vi "_easyXML_Marshal.vi"   [LabVIEW 2013, in "OpenSerializer.easyXML.lvlib"]
uses:
  OpenSerializer.easyXML.lvlib
  <vilib>/LabVIEW Open Source Project/OpenSerializer/Serializer/Serializer.lvclass
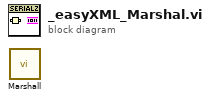
[diagram p0: block diagram]
diagram:
  n1 = call <vilib>:"Marshall.vi"() -> ()  [unwired: 9 in, 3 out]
